vi "Graph Circle.vi"() -> ()   [LabVIEW 2015]
panel:
  out "XY Circle Graph":cluster{dbl[], dbl[]}(graph)
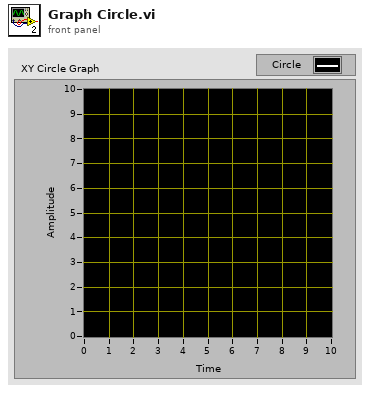
[diagram p1: front panel]
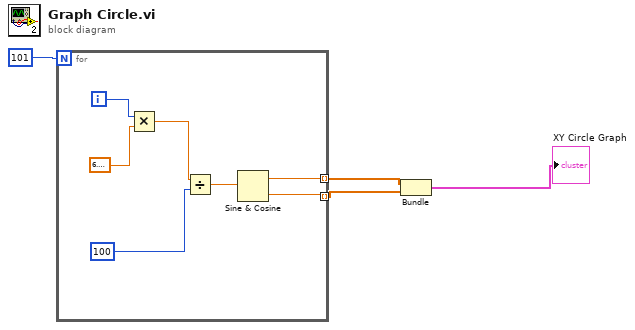
[diagram p0: block diagram]
diagram:
  n1 = for {
    N: 101 -> [_]
    tunnel: [w6] -> w3 mode=indexing
    tunnel: [w5] -> w2 mode=indexing
    i -> [w11]
    n2 = Multiply(x=w11, y=6.283185307179586) -> (x*y=w9:dbl)
    n3 = Divide(x=w9, y=100) -> (x/y=w7:dbl)
    n4 = Sine & Cosine(0:w7) -> (1:w6:dbl, 2:w5:dbl)
  }
  n5 = Bundle(w3, w2) -> (→"XY Circle Graph":cluster{dbl[], dbl[]})  [unwired: 1 in]
